vi "EyeSeeCam Plugin.vi"(10 "DC File":path, 11 "Data IN":T3={"Impulse Positions"=[{"Start"=395, "End"=549, "Impulse Plane"=enum."RALP", "Impulse Direction +ve?"=FALSE, "Time offset"=0, "Amplitude offset"=0.0}, {"Start"=603, "End"=760, "Impulse Plane"=enum."RALP", "Impulse Direction +ve?"=TRUE, "Time offset"=0, "Amplitude offset"=0.0}, {"Start"=785, "End"=938, "Impulse Plane"=enum."RALP", "Impulse Direction +ve?"=FALSE, "Time offset"=0, "Amplitude offset"=0.0}, {"Start"=980, "End"=1125, "Impulse Plane"=enum."LARP", "Impulse Direction +ve?"=FALSE, "Time offset"=0, "Amplitude offset"=0.0}, {"Start"=1179, "End"=1334, "Impulse Plane"=enum."LARP", "Impulse Direction +ve?"=TRUE, "Time offset"=0, "Amplitude offset"=0.0}, {"Start"=1723, "End"=1964, "Impulse Plane"=enum."Yaw", "Impulse Direction +ve?"=TRUE, "Time offset"=0, "Amplitude offset"=0.0}, {"Start"=1768, "End"=1968, "Impulse Plane"=enum."Yaw", "Impulse Direction +ve?"=TRUE, "Time offset"=0, "Amplitude offset"=0.0}, {"Start"=1812, "End"=1968, "Impulse Plane"=enum."Yaw", "Impulse Direction +ve?"=TRUE, "Time offset"=0, "Amplitude offset"=0.0}, {"Start"=4250, "End"=4393, "Impulse Plane"=enum."LARP", "Impulse Direction +ve?"=FALSE, "Time offset"=0, "Amplitude offset"=0.0}, {"Start"=4924, "End"=5072, "Impulse Plane"=enum."LARP", "Impulse Direction +ve?"=TRUE, "Time offset"=0, "Amplitude offset"=0.0}, {"Start"=5574, "End"=5721, "Impulse Plane"=enum."LARP", "Impulse Direction +ve?"=TRUE, "Time offset"=0, "Amplitude offset"=0.0}, {"Start"=6339, "End"=6491, "Impulse Plane"=enum."LARP", "Impulse Direction +ve?"=TRUE, "Time offset"=0, "Amplitude offset"=0.0}, {"Start"=6822, "End"=6967, "Impulse Plane"=enum."LARP", "Impulse Direction +ve?"=FALSE, "Time offset"=0, "Amplitude offset"=0.0}, {"Start"=7544, "End"=7701, "Impulse Plane"=enum."Pitch", "Impulse Direction +ve?"=TRUE, "Time offset"=0, "Amplitude offset"=0.0}, {"Start"=7928, "End"=8074, "Impulse Plane"=enum."LARP", "Impulse Direction +ve?"=TRUE, "Time offset"=0, "Amplitude offset"=0.0}, {"Start"=8313, "End"=8457, "Impulse Plane"=enum."LARP", "Impulse Direction +ve?"=FALSE, "Time offset"=0, "Amplitude offset"=0.0}, {"Start"=8807, "End"=8955, "Impulse Plane"=enum."LARP", "Impulse Direction +ve?"=FALSE, "Time offset"=0, "Amplitude offset"=0.0}, {"Start"=9308, "End"=9448, "Impulse Plane"=enum."LARP", "Impulse Direction +ve?"=FALSE, "Time offset"=0, "Amplitude offset"=0.0}, {"Start"=9758, "End"=9906, "Impulse Plane"=enum."LARP", "Impulse Direction +ve?"=TRUE, "Time offset"=0, "Amplitude offset"=0.0}, {"Start"=10165, "End"=10313, "Impulse Plane"=enum."LARP", "Impulse Direction +ve?"=TRUE, "Time offset"=0, "Amplitude offset"=0.0}, {"Start"=10605, "End"=10742, "Impulse Plane"=enum."LARP", "Impulse Direction +ve?"=FALSE, "Time offset"=0, "Amplitude offset"=0.0}, {"Start"=11345, "End"=11503, "Impulse Plane"=enum."Yaw", "Impulse Direction +ve?"=FALSE, "Time offset"=0, "Amplitude offset"=0.0}, {"Start"=12238, "End"=12394, "Impulse Plane"=enum."Yaw", "Impulse Direction +ve?"=FALSE, "Time offset"=0, "Amplitude offset"=0.0}, {"Start"=12374, "End"=12517, "Impulse Plane"=enum."LARP", "Impulse Direction +ve?"=FALSE, "Time offset"=0, "Amplitude offset"=0.0}, {"Start"=12860, "End"=13002, "Impulse Plane"=enum."LARP", "Impulse Direction +ve?"=TRUE, "Time offset"=0, "Amplitude offset"=0.0}, {"Start"=13499, "End"=13642, "Impulse Plane"=enum."LARP", "Impulse Direction +ve?"=FALSE, "Time offset"=0, "Amplitude offset"=0.0}, {"Start"=13998, "End"=14150, "Impulse Plane"=enum."LARP", "Impulse Direction +ve?"=TRUE, "Time offset"=0, "Amplitude offset"=0.0}, {"Start"=15617, "End"=15763, "Impulse Plane"=enum."LARP", "Impulse Direction +ve?"=FALSE, "Time offset"=0, "Amplitude offset"=0.0}], "No. Imp"=1, "Parameter Time Series"=[{"time offset"=0.0, "Offset"=0.0, "Gain"=1.0, "inverse"=FALSE, "filter data"=FALSE, "dots"=FALSE, "interpolate"=FALSE, "List 1"=1, "Color Box"=65295, "Boolean"=TRUE}, {"time offset"=0.0, "Offset"=0.0, "Gain"=1.0, "inverse"=FALSE, "filter data"=FALSE, "dots"=FALSE, "interpolate"=FALSE, "List 1"=13, "Color Box"=29695, "Boolean"=TRUE}], "Parameter Impuls Series"=[{"Color"=4652800, "Visible"=TRUE, "Channel"=7, "Invert"=FALSE, "Desaccade"=FALSE, "Offset"=0.0, "Gain"=1.0}, {"Color"=16860, "Visible"=TRUE, "Channel"=15, "Invert"=FALSE, "Desaccade"=FALSE, "Offset"=0.0, "Gain"=1.0}], "Experiment Parameters"={"Freq"=0.1, "Vel"=30, "Acc"=6000, "Stimulus"="HIT-RALP"}, "Autosort File"=refnum, "Data File"={"Data Channels"=array24x17202[412848 elements], "Sample Rate"=221, "Channel List"=["-", "Hz Velocity-in-Head", "-", "Hy Velocity-in-Head", "-", "Hx Velocity-in-Head", "Hl Velocity-in-Head", "Hr Velocity-in-Head", "-", "-", "-", "Lx Velocity-in-Head", "Ly Velocity-in-Head", "Lz Velocity-in-Head", "Ll Velocity-in-Head", "Lr Velocity-in-Head", "-", "-", "-", "Rx Velocity-in-Head", "Ry Velocity-in-Head", "Rz Velocity-in-Head", "Rl Velocity-in-Head", "Rr Velocity-in-Head"]}, "Experiment data path"=path "T:/50 _ HRC_DATA/Test Data/Vertical Canal VOG test", "Image data path"=path "C:/Users/w.figtree/Desktop", "LVS data path"=path "/Macintosh HD/Users/patrick/Studium/Diploma Thesis/Data Analysis", "Raw copy path"=path "/Macintosh HD/Users/patrick/Studium/Diploma Thesis/Data Analysis", "filename"="p00251s001e016c004t001.mat", "desaccading parameters"={"Tolerance"=3, "Acc Range"=7000.0, "Sample Rate"=221, "Impulse Plane 2"=enum."RALP", "Impulse dir"=TRUE}, "Experiment Parameters 2"={"Subject"="V Canal Test ", "Strain"="(2) _ vVOR", "Rotation plane"="YAW", "Experimenter"="Musterdoc", "Trial"=1.0, "Time"=8.0}, "Excel"={"Excel._Application"=refnum, "Use Excel"=TRUE, "Worksheet SINE"=refnum, "Row SINE"=0, "Worksheet TRANS"=refnum, "Row TRANS"=0}, "Session Config File"=refnum, "Autosort Parameter Set"=10, "EMA Version"="EMA 2011b", "desacc "={"Threshold 1 [Acc]"=7000.0, "Threshold 2 [% of TH1]"=60, "tolerance"=3, "Search WD "=0.1, " always use TH2"=FALSE, "Range"=3.0, "Max time"=120.0, "Min time"=20.0, "Velocity Threshold"=150}, "Cycle Nr for Saccades"={"POS"=0, "NEG"=3}, "calibration name"="No file selected"} {"Parameter Time Series"."time offset" format="%.3f"; "Parameter Time Series"."Gain" format="%.1f"; "Parameter Time Series"."Offset" format="%.1f"; "Parameter Time Series"."List 1" items=["Motor-Pos", "Motor-Vel", "Lx Position-in-Head", "Ly Position-in-Head", "Lz Position-in-Head", "Lx Velocity-in-Head", "Ly Velocity-in-Head", "Lz Velocity-in-Head", "Ll Velocity-in-Head", "Lr Velocity-in-Head", "Lx Accel-in-Head", "Ly Accel-in-Head", "Lz Accel-in-Head", "Rx Position-in-Head", "Ry Position-in-Head", "Rz Position-in-Head", "Rx Velocity-in-Head", "Ry Velocity-in-Head", "Rz Velocity-in-Head", "Rl Velocity-in-Head", "Rr Velocity-in-Head", "Rx Accel-in-Head", "Ry Accel-in-Head", "Rz Accel-in-Head", "Global Trigger", "", "", ""]; "Parameter Impuls Series"."Gain" format="%.1f"; "Parameter Impuls Series"."Offset" format="%.1f"}) -> (2 "Cancelled":bool, 3 "Data OUT":T3={"Impulse Positions"=[{"Start"=395, "End"=549, "Impulse Plane"=enum."RALP", "Impulse Direction +ve?"=FALSE, "Time offset"=0, "Amplitude offset"=0.0}, {"Start"=603, "End"=760, "Impulse Plane"=enum."RALP", "Impulse Direction +ve?"=TRUE, "Time offset"=0, "Amplitude offset"=0.0}, {"Start"=785, "End"=938, "Impulse Plane"=enum."RALP", "Impulse Direction +ve?"=FALSE, "Time offset"=0, "Amplitude offset"=0.0}, {"Start"=980, "End"=1125, "Impulse Plane"=enum."LARP", "Impulse Direction +ve?"=FALSE, "Time offset"=0, "Amplitude offset"=0.0}, {"Start"=1179, "End"=1334, "Impulse Plane"=enum."LARP", "Impulse Direction +ve?"=TRUE, "Time offset"=0, "Amplitude offset"=0.0}, {"Start"=1723, "End"=1964, "Impulse Plane"=enum."Yaw", "Impulse Direction +ve?"=TRUE, "Time offset"=0, "Amplitude offset"=0.0}, {"Start"=1768, "End"=1968, "Impulse Plane"=enum."Yaw", "Impulse Direction +ve?"=TRUE, "Time offset"=0, "Amplitude offset"=0.0}, {"Start"=1812, "End"=1968, "Impulse Plane"=enum."Yaw", "Impulse Direction +ve?"=TRUE, "Time offset"=0, "Amplitude offset"=0.0}, {"Start"=4250, "End"=4393, "Impulse Plane"=enum."LARP", "Impulse Direction +ve?"=FALSE, "Time offset"=0, "Amplitude offset"=0.0}, {"Start"=4924, "End"=5072, "Impulse Plane"=enum."LARP", "Impulse Direction +ve?"=TRUE, "Time offset"=0, "Amplitude offset"=0.0}, {"Start"=5574, "End"=5721, "Impulse Plane"=enum."LARP", "Impulse Direction +ve?"=TRUE, "Time offset"=0, "Amplitude offset"=0.0}, {"Start"=6339, "End"=6491, "Impulse Plane"=enum."LARP", "Impulse Direction +ve?"=TRUE, "Time offset"=0, "Amplitude offset"=0.0}, {"Start"=6822, "End"=6967, "Impulse Plane"=enum."LARP", "Impulse Direction +ve?"=FALSE, "Time offset"=0, "Amplitude offset"=0.0}, {"Start"=7544, "End"=7701, "Impulse Plane"=enum."Pitch", "Impulse Direction +ve?"=TRUE, "Time offset"=0, "Amplitude offset"=0.0}, {"Start"=7928, "End"=8074, "Impulse Plane"=enum."LARP", "Impulse Direction +ve?"=TRUE, "Time offset"=0, "Amplitude offset"=0.0}, {"Start"=8313, "End"=8457, "Impulse Plane"=enum."LARP", "Impulse Direction +ve?"=FALSE, "Time offset"=0, "Amplitude offset"=0.0}, {"Start"=8807, "End"=8955, "Impulse Plane"=enum."LARP", "Impulse Direction +ve?"=FALSE, "Time offset"=0, "Amplitude offset"=0.0}, {"Start"=9308, "End"=9448, "Impulse Plane"=enum."LARP", "Impulse Direction +ve?"=FALSE, "Time offset"=0, "Amplitude offset"=0.0}, {"Start"=9758, "End"=9906, "Impulse Plane"=enum."LARP", "Impulse Direction +ve?"=TRUE, "Time offset"=0, "Amplitude offset"=0.0}, {"Start"=10165, "End"=10313, "Impulse Plane"=enum."LARP", "Impulse Direction +ve?"=TRUE, "Time offset"=0, "Amplitude offset"=0.0}, {"Start"=10605, "End"=10742, "Impulse Plane"=enum."LARP", "Impulse Direction +ve?"=FALSE, "Time offset"=0, "Amplitude offset"=0.0}, {"Start"=11345, "End"=11503, "Impulse Plane"=enum."Yaw", "Impulse Direction +ve?"=FALSE, "Time offset"=0, "Amplitude offset"=0.0}, {"Start"=12238, "End"=12394, "Impulse Plane"=enum."Yaw", "Impulse Direction +ve?"=FALSE, "Time offset"=0, "Amplitude offset"=0.0}, {"Start"=12374, "End"=12517, "Impulse Plane"=enum."LARP", "Impulse Direction +ve?"=FALSE, "Time offset"=0, "Amplitude offset"=0.0}, {"Start"=12860, "End"=13002, "Impulse Plane"=enum."LARP", "Impulse Direction +ve?"=TRUE, "Time offset"=0, "Amplitude offset"=0.0}, {"Start"=13499, "End"=13642, "Impulse Plane"=enum."LARP", "Impulse Direction +ve?"=FALSE, "Time offset"=0, "Amplitude offset"=0.0}, {"Start"=13998, "End"=14150, "Impulse Plane"=enum."LARP", "Impulse Direction +ve?"=TRUE, "Time offset"=0, "Amplitude offset"=0.0}, {"Start"=15617, "End"=15763, "Impulse Plane"=enum."LARP", "Impulse Direction +ve?"=FALSE, "Time offset"=0, "Amplitude offset"=0.0}], "No. Imp"=1, "Parameter Time Series"=[{"time offset"=0.0, "Offset"=0.0, "Gain"=1.0, "inverse"=FALSE, "filter data"=FALSE, "dots"=FALSE, "interpolate"=FALSE, "List 1"=1, "Color Box"=65295, "Boolean"=TRUE}, {"time offset"=0.0, "Offset"=0.0, "Gain"=1.0, "inverse"=FALSE, "filter data"=FALSE, "dots"=FALSE, "interpolate"=FALSE, "List 1"=13, "Color Box"=29695, "Boolean"=TRUE}], "Parameter Impuls Series"=[{"Color"=4652800, "Visible"=TRUE, "Channel"=1, "Invert"=FALSE, "Desaccade"=FALSE, "Offset"=0.0, "Gain"=1.0}, {"Color"=16860, "Visible"=TRUE, "Channel"=13, "Invert"=FALSE, "Desaccade"=FALSE, "Offset"=0.0, "Gain"=1.0}], "Experiment Parameters"={"Freq"=0.1, "Vel"=30, "Acc"=6000, "Stimulus"="HIT-LARP"}, "Autosort File"=refnum, "Data File"={"Data Channels"=array24x20058[481392 elements], "Sample Rate"=221, "Channel List"=["-", "Hz Velocity-in-Head", "-", "Hy Velocity-in-Head", "-", "Hx Velocity-in-Head", "Hl Velocity-in-Head", "Hr Velocity-in-Head", "-", "-", "-", "Lx Velocity-in-Head", "Ly Velocity-in-Head", "Lz Velocity-in-Head", "Ll Velocity-in-Head", "Lr Velocity-in-Head", "-", "-", "-", "Rx Velocity-in-Head", "Ry Velocity-in-Head", "Rz Velocity-in-Head", "Rl Velocity-in-Head", "Rr Velocity-in-Head"]}, "Experiment data path"=path "T:/50 _ HRC_DATA/Test Data/Vertical Canal VOG test", "Image data path"=path "C:/Users/w.figtree/Desktop", "LVS data path"=path "/Macintosh HD/Users/patrick/Studium/Diploma Thesis/Data Analysis", "Raw copy path"=path "/Macintosh HD/Users/patrick/Studium/Diploma Thesis/Data Analysis", "filename"="p00251s001e016c005t001.mat", "desaccading parameters"={"Tolerance"=3, "Acc Range"=7000.0, "Sample Rate"=221, "Impulse Plane 2"=enum."RALP", "Impulse dir"=TRUE}, "Experiment Parameters 2"={"Subject"="V Canal Test ", "Strain"="(2) _ vVOR", "Rotation plane"="YAW", "Experimenter"="Musterdoc", "Trial"=1.0, "Time"=8.0}, "Excel"={"Excel._Application"=refnum, "Use Excel"=TRUE, "Worksheet SINE"=refnum, "Row SINE"=0, "Worksheet TRANS"=refnum, "Row TRANS"=0}, "Session Config File"=refnum, "Autosort Parameter Set"=10, "EMA Version"="EMA 2011b", "desacc "={"Threshold 1 [Acc]"=7000.0, "Threshold 2 [% of TH1]"=60, "tolerance"=3, "Search WD "=0.1, " always use TH2"=FALSE, "Range"=3.0, "Max time"=120.0, "Min time"=20.0, "Velocity Threshold"=150}, "Cycle Nr for Saccades"={"POS"=0, "NEG"=3}, "calibration name"="No file selected"} {"Parameter Time Series"."time offset" format="%.3f"; "Parameter Time Series"."Gain" format="%.1f"; "Parameter Time Series"."Offset" format="%.1f"; "Parameter Time Series"."List 1" items=["Motor-Pos", "Motor-Vel", "Lx Position-in-Head", "Ly Position-in-Head", "Lz Position-in-Head", "Lx Velocity-in-Head", "Ly Velocity-in-Head", "Lz Velocity-in-Head", "Ll Velocity-in-Head", "Lr Velocity-in-Head", "Lx Accel-in-Head", "Ly Accel-in-Head", "Lz Accel-in-Head", "Rx Position-in-Head", "Ry Position-in-Head", "Rz Position-in-Head", "Rx Velocity-in-Head", "Ry Velocity-in-Head", "Rz Velocity-in-Head", "Rl Velocity-in-Head", "Rr Velocity-in-Head", "Rx Accel-in-Head", "Ry Accel-in-Head", "Rz Accel-in-Head", "Global Trigger", "", "", ""]; "Parameter Impuls Series"."Gain" format="%.1f"; "Parameter Impuls Series"."Offset" format="%.1f"})   [LabVIEW 2016]
uses:
  core/type-defs/TD_Statemachine-Data.ctl
  core/type-defs/TD_Time Series.ctl
  core/type-defs/TD_Impulse Parameter.ctl
  core/core.lvlib
panel:
  out "Process Error":errorcluster
  in  "BTN_Process":bool
  in  "Tab Control":enum32{"Settings", "Time Plot", "Impulse Plot"}(tab)
  in  "Btn_ZeroGyro":bool
  in  "alignPR?":bool caption="Align Head pitch/roll axes?"
  in  "manualGOff?":bool caption="Use manual gyro offset?"
  in  "Yaw":dbl caption="Yaw (dps)"
  in  "Pitch":dbl caption="Pitch (dps)"
  in  "Roll":dbl caption="Roll (dps)"
  in  "Head Calibration File":path
  in  "Data File":path
  in  "Eye Calibration File":path
  in  "eyeFromPx?":bool=TRUE caption="Calculate eye data from pupil centroid?"
  in  "Time Plot Selection":T1=[{"time offset"=0.0, "Offset"=0.0, "Gain"=1.0, "inverse"=FALSE, "filter data"=FALSE, "dots"=FALSE, "interpolate"=FALSE, "List 1"=1, "Color Box"=65295, "Boolean"=TRUE}, {"time offset"=0.0, "Offset"=0.0, "Gain"=1.0, "inverse"=FALSE, "filter data"=FALSE, "dots"=FALSE, "interpolate"=FALSE, "List 1"=3, "Color Box"=16717731, "Boolean"=FALSE}, {"time offset"=0.0, "Offset"=0.0, "Gain"=1.0, "inverse"=FALSE, "filter data"=FALSE, "dots"=FALSE, "interpolate"=FALSE, "List 1"=6, "Color Box"=16742144, "Boolean"=FALSE}, {"time offset"=0.0, "Offset"=0.0, "Gain"=1.0, "inverse"=FALSE, "filter data"=FALSE, "dots"=FALSE, "interpolate"=FALSE, "List 1"=7, "Color Box"=14419712, "Boolean"=FALSE}, {"time offset"=0.0, "Offset"=0.0, "Gain"=1.0, "inverse"=FALSE, "filter data"=FALSE, "dots"=FALSE, "interpolate"=FALSE, "List 1"=13, "Color Box"=16777224, "Boolean"=TRUE}, {"time offset"=0.0, "Offset"=0.0, "Gain"=1.0, "inverse"=FALSE, "filter data"=FALSE, "dots"=FALSE, "interpolate"=FALSE, "List 1"=12, "Color Box"=2298623, "Boolean"=FALSE}] {"time offset" format="%.3f"; "Gain" format="%.1f"; "Offset" format="%.1f"; "List 1" items=["-", "Hz Velocity-in-Head", "-", "Hy Velocity-in-Head", "-", "Hx Velocity-in-Head", "Hl Velocity-in-Head", "Hr Velocity-in-Head", "-", "Ly Position-in-Head", "Lz Position-in-Head", "-", "Ly Velocity-in-Head", "Lz Velocity-in-Head", "-", "-", "-", "-", "-", "-", "-", "-", "-", "-"]}
  in  "Impulse Plot Selection":T2=[{"Color"=4652800, "Visible"=TRUE, "Channel"=1, "Invert"=FALSE, "Desaccade"=FALSE, "Offset"=0.0, "Gain"=1.0}, {"Color"=16717731, "Visible"=FALSE, "Channel"=3, "Invert"=FALSE, "Desaccade"=FALSE, "Offset"=0.0, "Gain"=1.0}, {"Color"=16742144, "Visible"=FALSE, "Channel"=6, "Invert"=FALSE, "Desaccade"=FALSE, "Offset"=0.0, "Gain"=1.0}, {"Color"=14419712, "Visible"=FALSE, "Channel"=7, "Invert"=FALSE, "Desaccade"=FALSE, "Offset"=0.0, "Gain"=1.0}, {"Color"=16777224, "Visible"=TRUE, "Channel"=13, "Invert"=FALSE, "Desaccade"=FALSE, "Offset"=0.0, "Gain"=1.0}, {"Color"=2298623, "Visible"=FALSE, "Channel"=12, "Invert"=FALSE, "Desaccade"=FALSE, "Offset"=0.0, "Gain"=1.0}] {"Gain" format="%.1f"; "Offset" format="%.1f"; "Channel" items=["-", "Hz Velocity-in-Head", "-", "Hy Velocity-in-Head", "-", "Hx Velocity-in-Head", "Hl Velocity-in-Head", "Hr Velocity-in-Head", "-", "Ly Position-in-Head", "Lz Position-in-Head", "-", "Ly Velocity-in-Head", "Lz Velocity-in-Head", "-", "-", "-", "-", "-", "-", "-", "-", "-", "-"]}
  # "Specify a file for analysis..."
  # "Offset    Gain       Inv                     Channel                       Col   Vis  Sac"
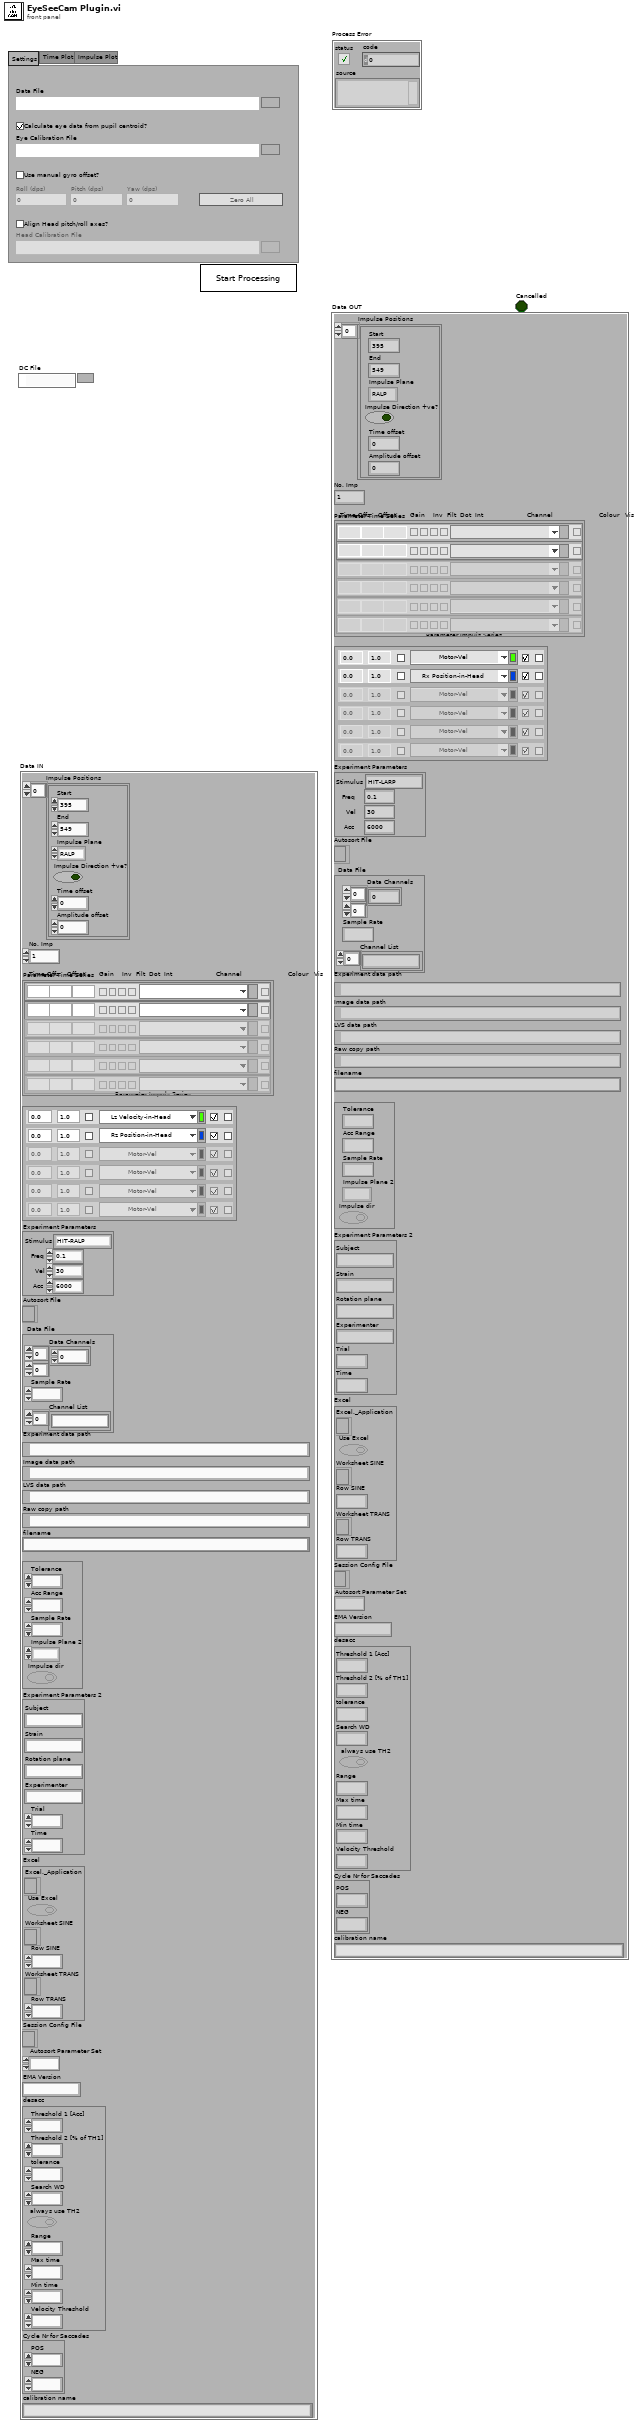
[diagram p1: front panel]
types:
  T1 = typedef "core.lvlib/TD_Time Series.ctl" = cluster{"time offset":dbl, "Offset":dbl, "Gain":dbl, "inverse":bool, "filter data":bool, "dots":bool, "interpolate":bool, "List 1":u16, "Color Box":u32, "Boolean":bool}[]
  T2 = typedef "core.lvlib/TD_Impulse Parameter.ctl" = cluster{"Color":u32, "Visible":bool, "Channel":u16, "Invert":bool, "Desaccade":bool, "Offset":dbl, "Gain":dbl}[]
  T3 = typedef "core.lvlib/TD_Statemachine-Data.ctl" = cluster{"Impulse Positions":cluster{"Start":i32, "End":i32, "Impulse Plane":enum16{"Other", "Yaw", "Pitch", "Roll", "LARP", "RALP"}, "Impulse Direction +ve?":bool, "Time offset":i32, "Amplitude offset":dbl}[], "No. Imp":i32, "Parameter Time Series":T1, "Parameter Impuls Series":T2, "Experiment Parameters":cluster{"Freq":dbl, "Vel":i32, "Acc":i32, "Stimulus":string}, "Autosort File":refnum<file>, "Data File":cluster{"Data Channels":dbl[][], "Sample Rate":i32, "Channel List":string[]}, "Experiment data path":path, "Image data path":path, "LVS data path":path, "Raw copy path":path, "filename":string, "desaccading parameters":cluster{"Tolerance":i32, "Acc Range":dbl, "Sample Rate":i32, "Impulse Plane 2":enum16{"Other", "Yaw", "Pitch", "Roll", "LARP", "RALP"}, "Impulse dir":bool}, "Experiment Parameters 2":cluster{"Subject":string, "Strain":string, "Rotation plane":string, "Experimenter":string, "Trial":dbl, "Time":dbl}, "Excel":cluster{"Excel._Application":refnum<k7>, "Use Excel":bool, "Worksheet SINE":refnum<k7>, "Row SINE":i32, "Worksheet TRANS":refnum<k7>, "Row TRANS":i32}, "Session Config File":refnum<file>, "Autosort Parameter Set":i32, "EMA Version":string, "desacc ":cluster{"Threshold 1 [Acc]":dbl, "Threshold 2 [% of TH1]":i32, "tolerance":i32, "Search WD ":dbl, " always use TH2":bool, "Range":dbl, "Max time":dbl, "Min time":dbl, "Velocity Threshold":i32}, "Cycle Nr for Saccades":cluster{"POS":i32, "NEG":i32}, "calibration name":string}
  T4 = enum8{"Enabled", "Disabled", "Disabled and Grayed Out"}
  T5 = cluster{"time offset":dbl, "Offset":dbl, "Gain":dbl, "inverse":bool, "filter data":bool, "dots":bool, "interpolate":bool, "List 1":u16, "Color Box":u32, "Boolean":bool}
  T6 = cluster{"Color":u32, "Visible":bool, "Channel":u16, "Invert":bool, "Desaccade":bool, "Offset":dbl, "Gain":dbl}
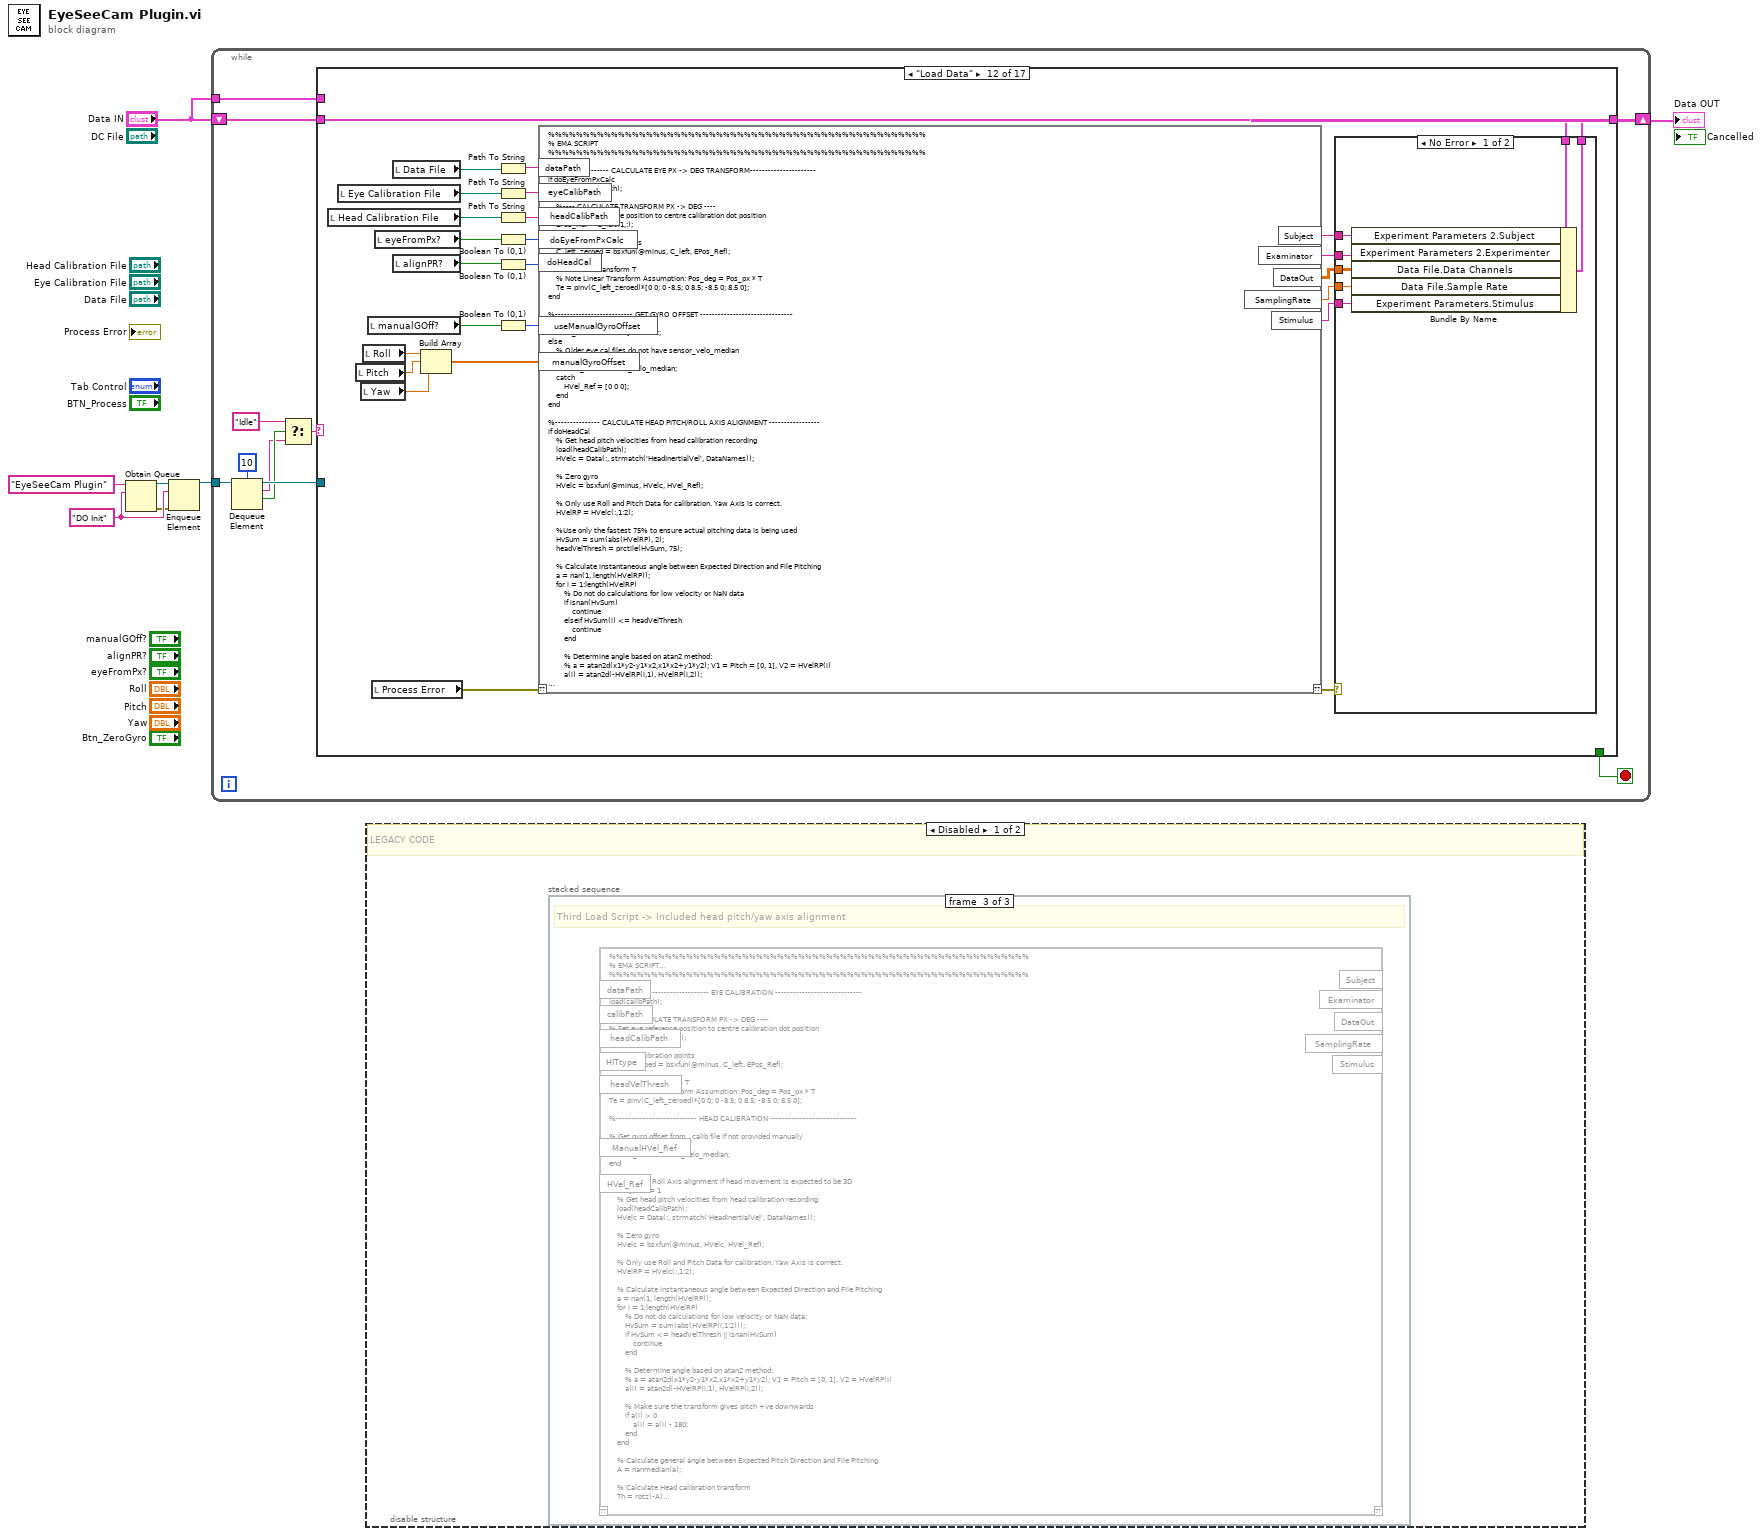
[diagram p0: block diagram]
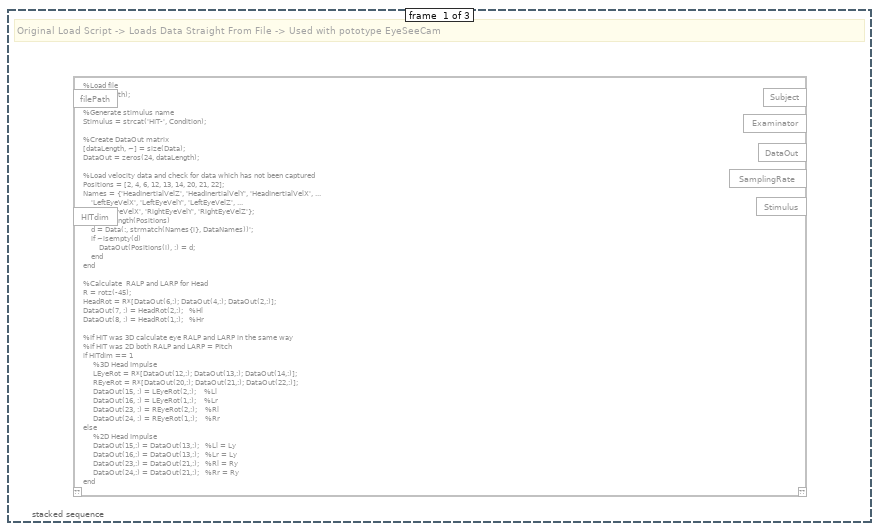
[diagram p2: hidden frame]
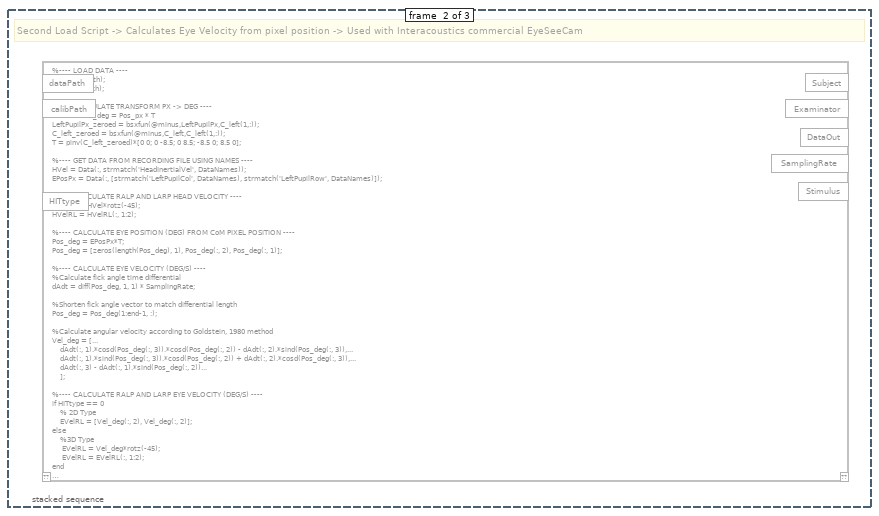
[diagram p3: hidden frame]
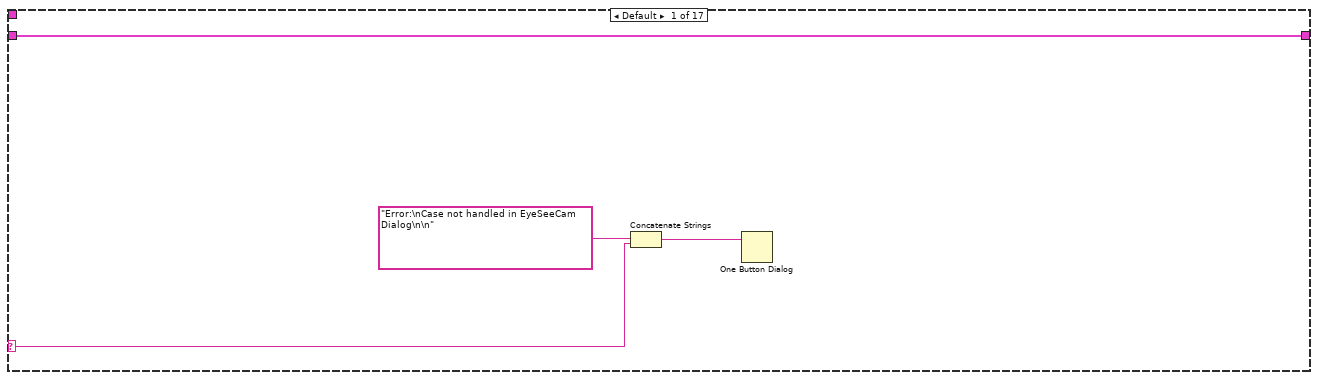
[diagram p5: hidden frame]
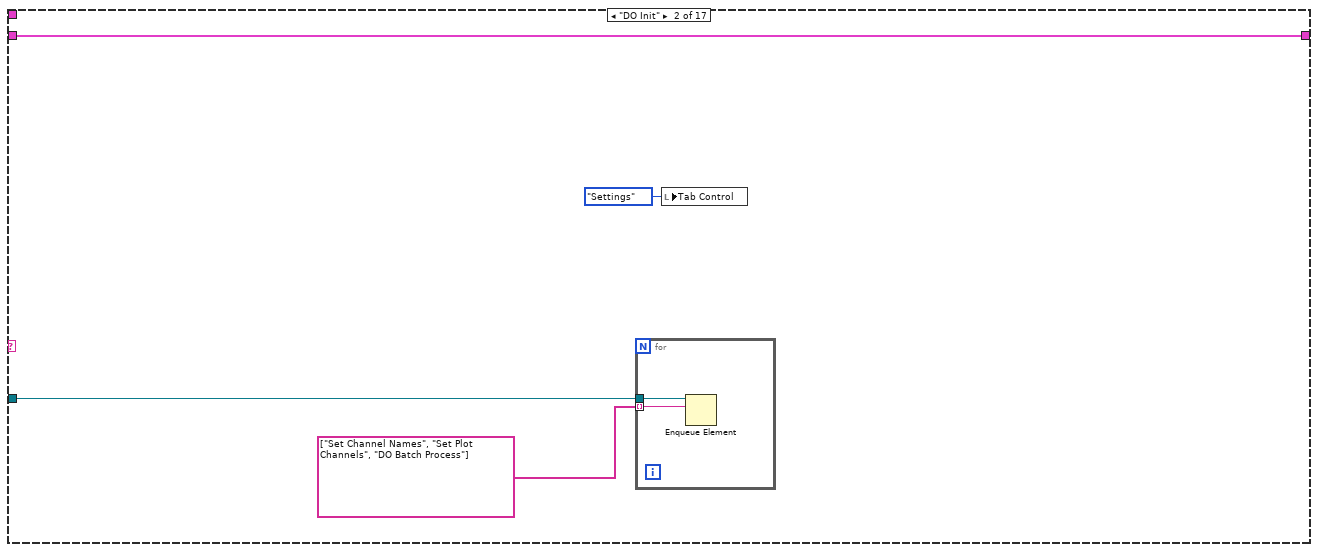
[diagram p6: hidden frame]
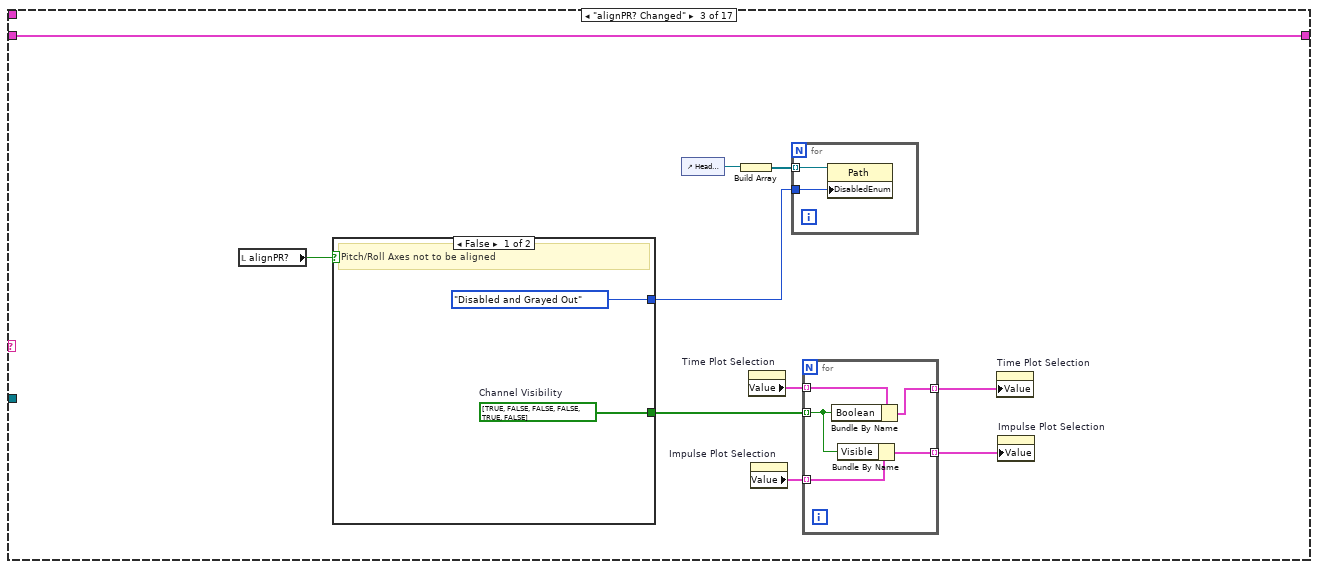
[diagram p7: hidden frame]
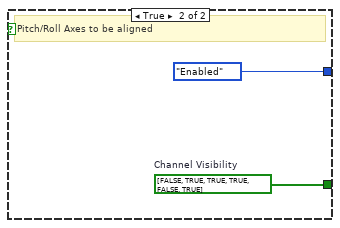
[diagram p8: hidden frame]
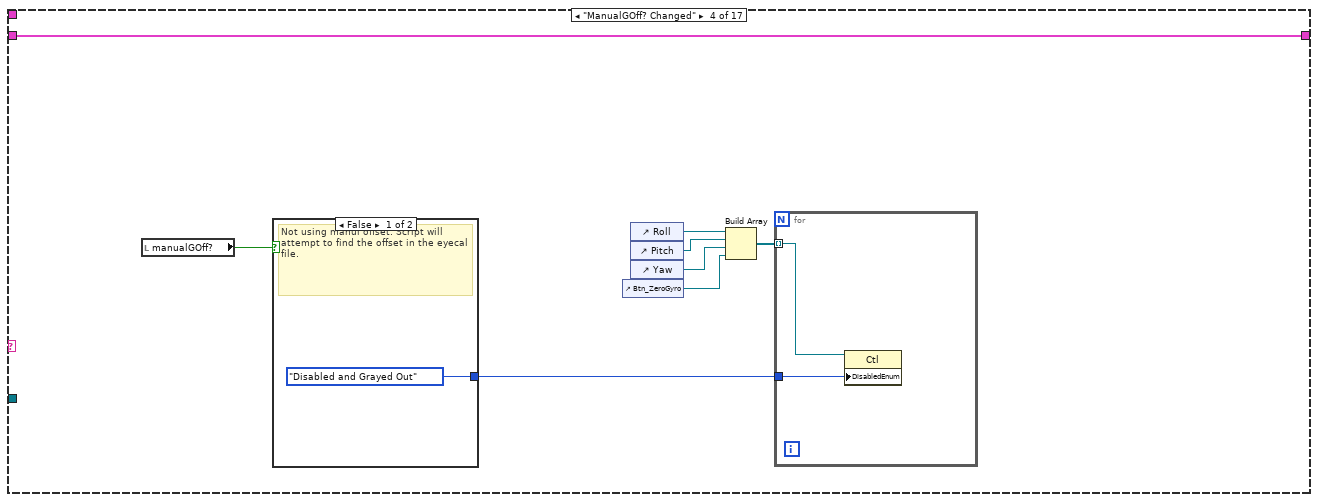
[diagram p9: hidden frame]
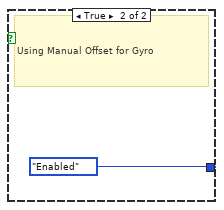
[diagram p10: hidden frame]
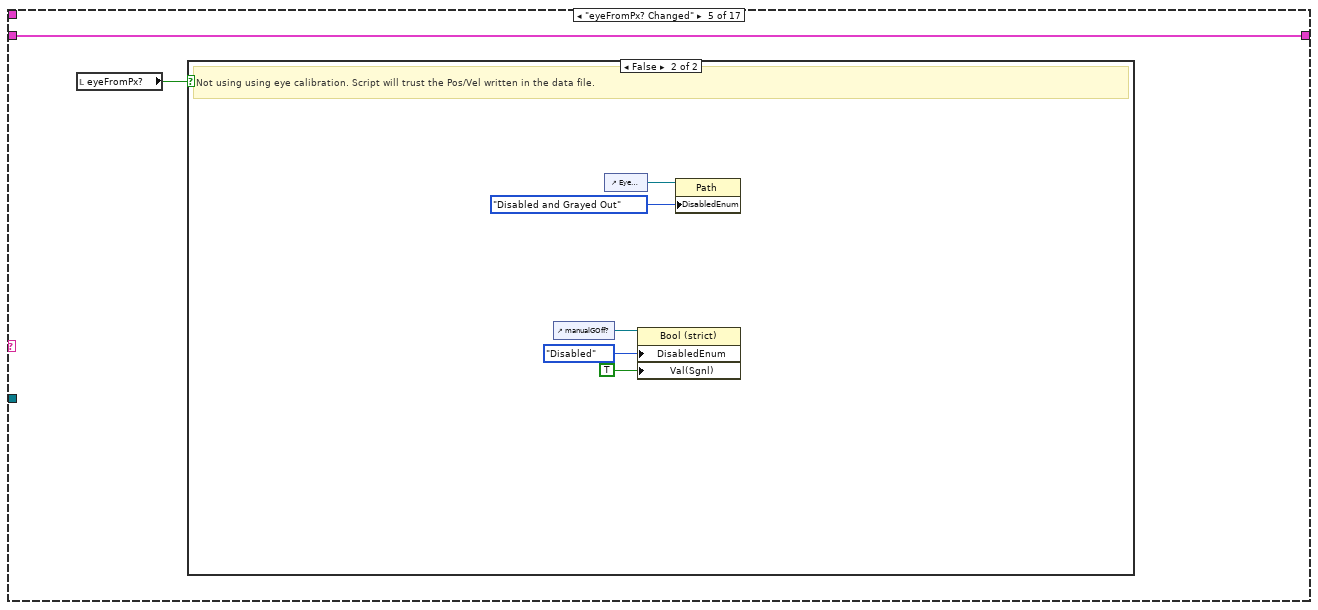
[diagram p11: hidden frame]
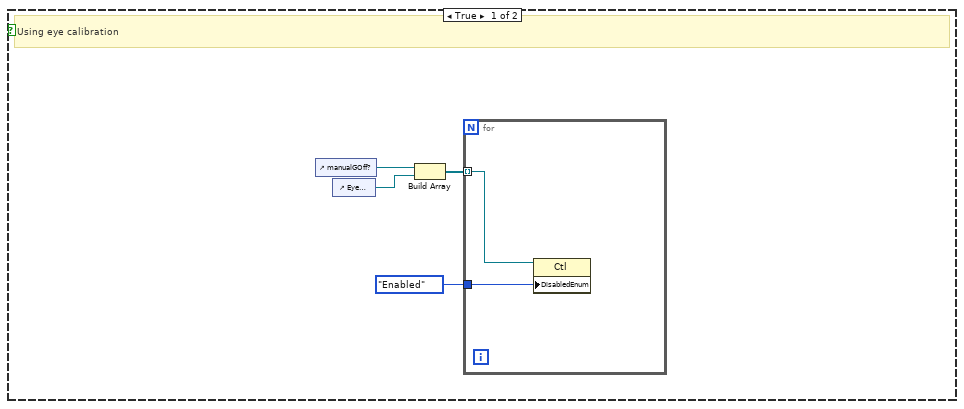
[diagram p12: hidden frame]
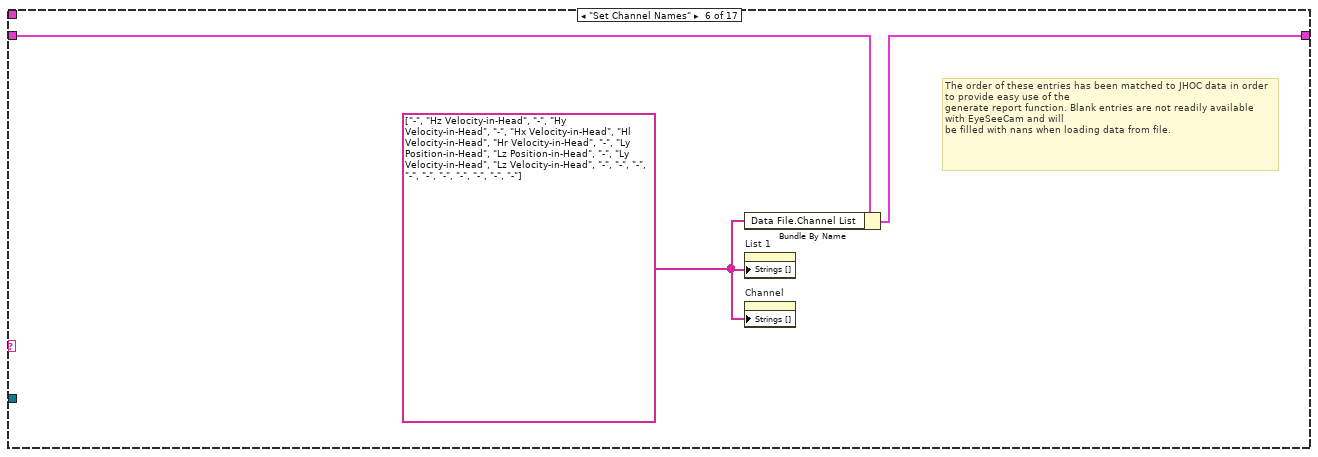
[diagram p13: hidden frame]
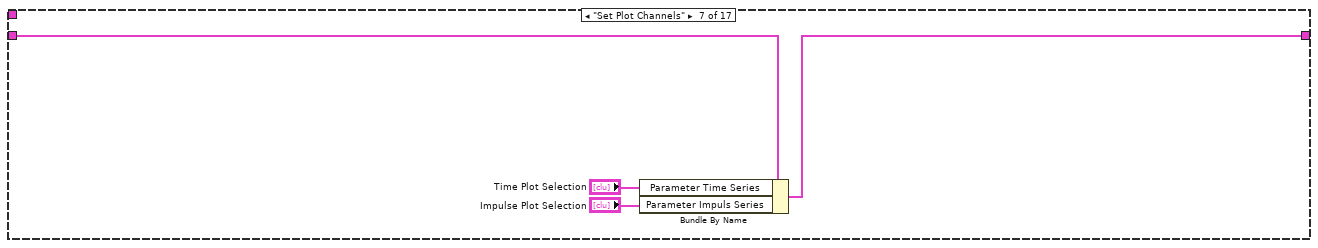
[diagram p14: hidden frame]
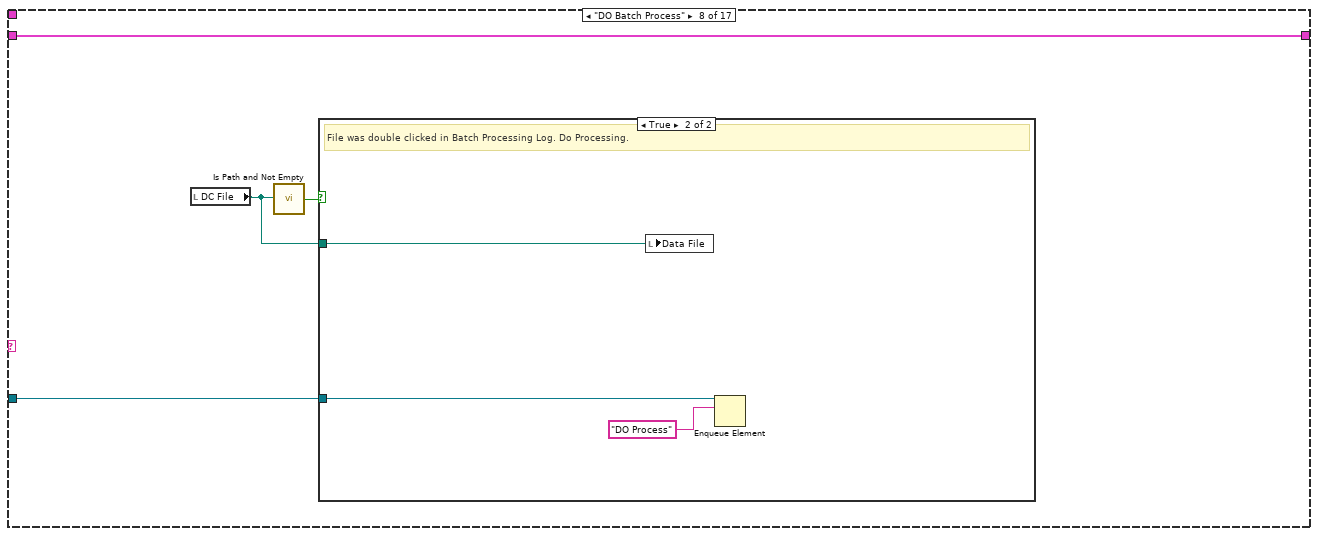
[diagram p15: hidden frame]
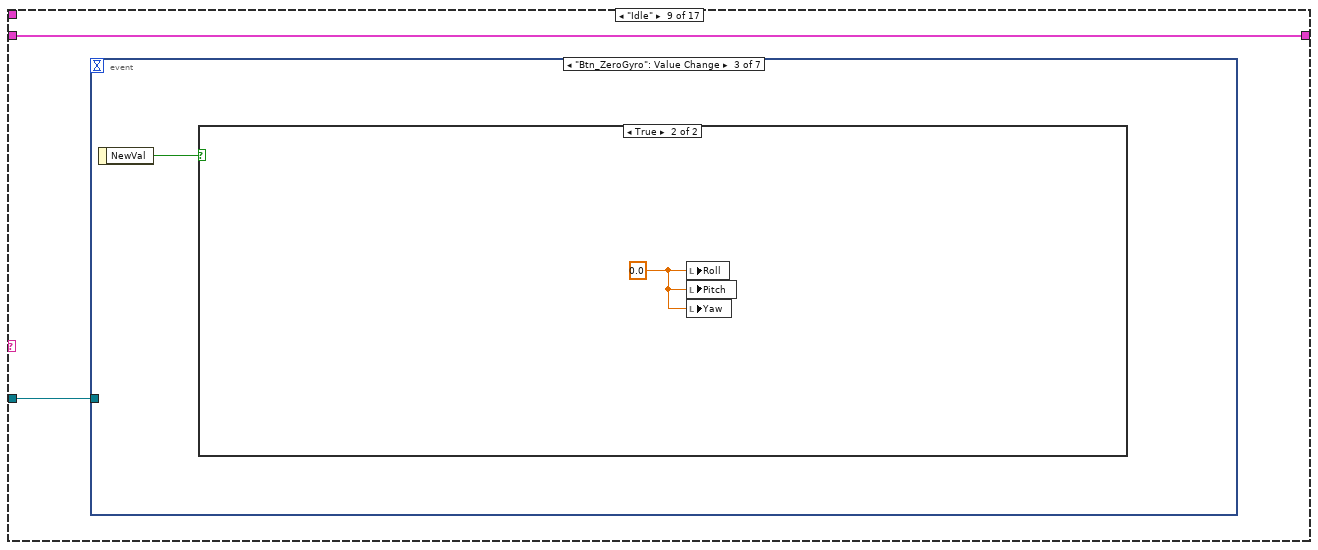
[diagram p17: hidden frame]
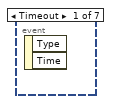
[diagram p18: hidden frame]
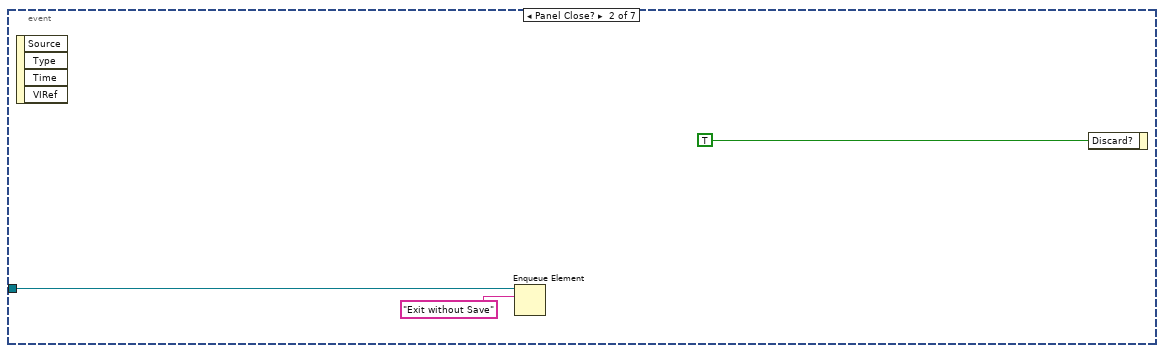
[diagram p19: hidden frame]
diagram:
  w5 = "DO Init" ("name (unnamed)")
  n1 = Obtain Queue(name (unnamed)="EyeSeeCam Plugin", element data type=w5) -> (queue out=w6:refnum<queue>, error out=w4:errorcluster)  [unwired: 3 in, 1 out]
  n2 = Enqueue Element(queue=w6, element=w5, error in (no error)=w4) -> (queue out=w3:refnum<queue>)  [unwired: 1 in, 2 out]
  n3 = while {
    tunnel: w3 -> [w18]
    shift-right: [w16] -> w2
    shift-left: "Data IN" -> [w17]
    tunnel: "Data IN" -> [w13]
    stop <- w14 stop-if-true
    n4 = Dequeue Element(queue=w18, timeout in ms (-1)=10) -> (queue out=w15:refnum<queue>, element=w11:string, timed out?=w12:bool)  [unwired: 1 in, 1 out]
    n5 = Select(t="Idle", s=w12, f=w11) -> (s? t:f=w9:string)
    n6 = case shown="\"Load Data\"" w9 {
      selector: w9 -> [w20 _ _ _ _ _ _ _ _ _ _ _ _ _ _ _ _]
      tunnel: w17 -> [w22 w26 w38 w57 w63 w77 w81 w84 w90 w109 w113 w137 w164 w178 w181 w197 _]
      tunnel: [w22 w26 w38 w57 w63 w76 w80 w84 w90 w109 w113 w136 w163 w178 w181 w197 w201] -> w16
      tunnel: w15 -> [_ w25 _ _ _ _ _ w85 w89 w108 _ _ _ w174 _ _ _]
      tunnel: [_ _ _ _ _ _ _ _ _ _ _ _ _ _ _ TRUE TRUE] -> w14
      tunnel: w13 -> [_ _ _ _ _ _ _ _ _ _ _ _ _ _ _ _ w201]
      frame Default {
        n7 = Concatenate Strings("Error:\nCase not handled in EyeSeeCam Dialog\n\n" ("message"), w20) -> (w19:string)
        n8 = One Button Dialog(message=w19) -> ()  [unwired: 1 in, 1 out]
      }
      frame "DO Init" {
        n9 = for {
          tunnel: w25 -> [w28]
          tunnel: string[] ["Set Channel Names", "Set Plot Channels", "DO Batch Process"] -> [w27] mode=indexing
          n10 = Enqueue Element(queue=w28, element=w27) -> ()  [unwired: 2 in, 3 out]
        }
        n11 = local write "Tab Control"(enum32{"Settings", "Time Plot", "Impulse Plot"}."Settings" ("Tab Control")) -> ()
      }
      frame "alignPR? Changed" {
        n12 = local read "alignPR?"() -> (w37:bool)
        n13 = case shown="False" w37 {
          tunnel: [T4."Disabled and Grayed Out" ("Disabled") T4."Enabled" ("Disabled")] -> w29
          tunnel: [w46 w48] -> w35
          frame False {
            w46 = bool[] [TRUE, FALSE, FALSE, FALSE, TRUE, FALSE]  # Channel Visibility
            # "Pitch/Roll Axes not to be aligned"
          }
          frame True {
            w48 = bool[] [FALSE, TRUE, TRUE, TRUE, FALSE, TRUE]  # Channel Visibility
            # "Pitch/Roll Axes to be aligned"
          }
        }
        n14 = control-ref of="Head Calibration File"() -> (w31:refnum<vi>)
        n15 = Build Array(w31) -> (w30:refnum<vi>[])
        n16 = property on="Time Plot Selection" class="Arr (strict)"() -> ("Value"=w36:T1)  [unwired: 2 in, 2 out]
        n17 = property on="Impulse Plot Selection" class="Arr (strict)"() -> ("Value"=w33:T2)  [unwired: 2 in, 2 out]
        n18 = for {
          tunnel: w30 -> [w40] mode=indexing
          tunnel: w29 -> [w39]
          n19 = property class="Path"(reference=w40, "DisabledEnum"=w39) -> ()  [unwired: 1 in, 2 out]
        }
        n20 = for {
          tunnel: w36 -> [w45] mode=indexing
          tunnel: [w44] -> w34 mode=indexing
          tunnel: w35 -> [w41] mode=indexing
          tunnel: w33 -> [w43] mode=indexing
          tunnel: [w42] -> w32 mode=indexing
          n21 = Bundle By Name(cluster=w45, "Boolean"=w41) -> (w44:T5)
          n22 = Bundle By Name(cluster=w43, "Visible"=w41) -> (w42:T6)
        }
        n23 = property on="Time Plot Selection" class="Arr (strict)"("Value"=w34) -> ()  [unwired: 2 in, 2 out]
        n24 = property on="Impulse Plot Selection" class="Arr (strict)"("Value"=w32) -> ()  [unwired: 2 in, 2 out]
      }
      frame "ManualGOff? Changed" {
        n25 = local read "manualGOff?"() -> (w56:bool)
        n26 = case shown="False" w56 {
          tunnel: [T4."Disabled and Grayed Out" ("Disabled") T4."Enabled" ("Disabled")] -> w51
          frame False {
            # "Not using manul offset. Script will attempt to find the offset in the eyecal file."
          }
          frame True {
            # "Using Manual Offset for Gyro"
          }
        }
        n27 = control-ref of="Btn_ZeroGyro"() -> (w50:refnum<vi>)
        n28 = control-ref of="Roll"() -> (w55:refnum<vi>)
        n29 = control-ref of="Pitch"() -> (w54:refnum<vi>)
        n30 = control-ref of="Yaw"() -> (w53:refnum<vi>)
        n31 = Build Array(w55, w54, w53, w50) -> (w52:refnum<vi>[])
        n32 = for {
          tunnel: w52 -> [w59] mode=indexing
          tunnel: w51 -> [w58]
          n33 = property class="Ctl"(reference=w59, "DisabledEnum"=w58) -> ()  [unwired: 1 in, 2 out]
        }
      }
      frame "eyeFromPx? Changed" {
        n34 = local read "eyeFromPx?"() -> (w62:bool)
        n35 = case shown="False" w62 {
          frame True {
            # "Using eye calibration"
            n36 = control-ref of="manualGOff?"() -> (w66:refnum<vi>)
            n37 = control-ref of="Eye Calibration File"() -> (w65:refnum<vi>)
            n38 = Build Array(w66, w65) -> (w67:refnum<vi>[])
            n39 = for {
              tunnel: w67 -> [w69] mode=indexing
              tunnel: T4."Enabled" ("Disabled") -> [w68]
              n40 = property class="Ctl"(reference=w69, "DisabledEnum"=w68) -> ()  [unwired: 1 in, 2 out]
            }
          }
          frame False {
            # "Not using using eye calibration. Script will trust the Pos/Vel written in the data file."
            n41 = control-ref of="manualGOff?"() -> (w72:refnum<vi>)
            n42 = control-ref of="Eye Calibration File"() -> (w73:refnum<vi>)
            n43 = property class="Bool (strict)"(reference=w72, "DisabledEnum"=T4."Disabled" ("Disabled"), "Val(Sgnl)"=TRUE ("Value")) -> ()  [unwired: 1 in, 2 out]
            n44 = property class="Path"(reference=w73, "DisabledEnum"=T4."Disabled and Grayed Out" ("Disabled")) -> ()  [unwired: 1 in, 2 out]
          }
        }
      }
      frame "Set Channel Names" {
        w75 = string[] ["-", "Hz Velocity-in-Head", "-", "Hy Velocity-in-Head", "-", "Hx Velocity-in-Head", "Hl Velocity-in-Head", "Hr Velocity-in-Head", "-", "Ly Position-in-Head", "Lz Position-in-Head", "-", "Ly Velocity-in-Head", "Lz Velocity-in-Head", "-", "-", "-", "-", "-", "-", "-", "-", "-", "-"]
        # "The order of these entries has been matched to JHOC data in order to provide easy use of the\ngenerate report function. Blank entries are not readily available with EyeSeeCam and will\nbe filled with nans when loading data from file."
        n45 = Bundle By Name(cluster=w77, "Data File.Channel List"=w75) -> (w76:T3)
        n46 = property on="List 1" class="Ring (strict)"("Strings []"=w75) -> ()  [unwired: 2 in, 2 out]
        n47 = property on="Channel" class="Ring (strict)"("Strings []"=w75) -> ()  [unwired: 2 in, 2 out]
      }
      frame "Set Plot Channels" {
        n48 = Bundle By Name(cluster=w81, "Parameter Time Series"="Time Plot Selection", "Parameter Impuls Series"="Impulse Plot Selection") -> (w80:T3)
      }
      frame "DO Batch Process" {
        n49 = local read "DC File"() -> (w83:path)
        n50 = call <vilib>:"Is Path and Not Empty.vi"("path"=w83) -> ("Is Path and Not Empty?"=w82:bool)  [unwired: 4 in]
        n51 = case shown="True" w82 {
          tunnel: w83 -> [_ w88]
          tunnel: w85 -> [_ w87]
          frame False {
            # "This dialog was not open by batch processing. Do nothing."
          }
          frame True {
            # "File was double clicked in Batch Processing Log. Do Processing."
            n52 = local write "Data File"(w88) -> ()
            n53 = Enqueue Element(queue=w87, element="DO Process") -> ()  [unwired: 2 in, 3 out]
          }
        }
      }
      frame "Idle" {
        n54 = event shown="[2] \"Btn_ZeroGyro\": Value Change" {
          selector: _ -> [_ _ _ _ _ _ _]
          dyn-events: _ -> [_ _ _ _ _ _ _]
          timeout: _ -> [_ _ _ _ _ _ _]
          tunnel: w89 -> [_ w91 _ w97 w98 w103 w105]
          event Timeout {
            n55 = event-data() -> ()  [unwired: 1 in, 2 out]
          }
          event Panel Close? {
            n56 = event-data() -> ()  [unwired: 1 in, 4 out]
            n57 = Enqueue Element(queue=w91, element="Exit without Save") -> ()  [unwired: 2 in, 3 out]
            n58 = event-data("Discard?"=TRUE) -> ()  [unwired: 1 in, 1 out]
          }
          event "Btn_ZeroGyro": Value Change {
            n59 = event-data() -> ("NewVal"=w94:bool)  [unwired: 1 in]
            n60 = case shown="True" w94 {
              frame False {
              }
              frame True {
                w95 = 0.0 ("Roll")
                n61 = local write "Roll"(w95) -> ()
                n62 = local write "Pitch"(w95) -> ()
                n63 = local write "Yaw"(w95) -> ()
              }
            }
          }
          event "BTN_Process": Mouse Down {
            n64 = event-data() -> ()  [unwired: 1 in, 7 out]
            n65 = Enqueue Element(queue=w97, element="DO Process") -> ()  [unwired: 2 in, 3 out]
          }
          event "eyeFromPx?": Value Change {
            n66 = event-data() -> ()  [unwired: 1 in, 6 out]
            n67 = Enqueue Element(queue=w98, element="eyeFromPx? Changed") -> ()  [unwired: 2 in, 3 out]
          }
          event "alignPR?": Value Change {
            n68 = event-data() -> ()  [unwired: 1 in, 6 out]
            n69 = Enqueue Element(queue=w103, element="alignPR? Changed") -> (queue out=w101:refnum<queue>)  [unwired: 2 in, 2 out]
            n70 = Enqueue Element(queue=w101, element="Set Plot Channels") -> ()  [unwired: 2 in, 3 out]
          }
          event "manualGOff?": Value Change {
            n71 = event-data() -> ()  [unwired: 1 in, 6 out]
            n72 = Enqueue Element(queue=w105, element="ManualGOff? Changed") -> ()  [unwired: 2 in, 3 out]
          }
        }
      }
      frame "DO Process" {
        # "Clear Processing Errors"
        n73 = for {
          tunnel: w108 -> [w111]
          tunnel: string[] ["Check Files", "Load Data", "Get File Info", "Report Errors"] -> [w110] mode=indexing
          n74 = Enqueue Element(queue=w111, element=w110) -> ()  [unwired: 2 in, 3 out]
        }
        n75 = local write "Process Error"(errorcluster {"status"=FALSE, "code"=0, "source"=""} ("Process Error")) -> ()
      }
      frame "Check Files" {
        n76 = local read "Process Error"() -> (w112:errorcluster)
        n77 = case shown="No Error" w112 {
          frame No Error {
            # "Only require head calibration  file when head calibration is selected"
            # "Only require eye calibration file when eye calibration is selected"
            # "Always require data file"
            n78 = local read "Head Calibration File"() -> (w123:path)
            n79 = local read "Eye Calibration File"() -> (w124:path)
            n80 = local read "Data File"() -> (w125:path)
            n81 = local read "eyeFromPx?"() -> (w122:bool)
            n82 = local read "alignPR?"() -> (w120:bool)
            n83 = call <vilib>:"Is Path and Not Empty.vi"("path"=w125) -> ("Is Path and Not Empty?"=w118:bool)  [unwired: 4 in]
            n84 = call <vilib>:"Is Path and Not Empty.vi"("path"=w123) -> ("Is Path and Not Empty?"=w119:bool)  [unwired: 4 in]
            n85 = call <vilib>:"Is Path and Not Empty.vi"("path"=w124) -> ("Is Path and Not Empty?"=w121:bool)  [unwired: 4 in]
            n86 = Compound Arithmetic op=OR(invert w120, w119) -> (w116:bool)
            n87 = Compound Arithmetic op=OR(invert w122, w121) -> (w117:bool)
            n88 = Compound Arithmetic op=AND(w118, w117, w116) -> (w115:bool)
            n89 = case shown="False" w115 {
              tunnel: [errorcluster {"status"=TRUE, "code"=0, "source"="Files must be specified for each selected file field."} ("error constant") _] -> w114
              frame False {
                # "File requirements not met. Error."
              }
              frame True {
                # "All file requirments met."
              }
            }
            n90 = local write "Process Error"(w114) -> ()
          }
          frame Error {
          }
        }
      }
      frame "Load Data" {
        n91 = local read "Head Calibration File"() -> (w149:path)
        n92 = local read "Eye Calibration File"() -> (w150:path)
        n93 = local read "Pitch"() -> (w146:dbl)
        n94 = local read "Yaw"() -> (w145:dbl)
        n95 = local read "Roll"() -> (w147:dbl)
        n96 = local read "manualGOff?"() -> (w148:bool)
        n97 = local read "Process Error"() -> (w138:errorcluster)
        n98 = local read "eyeFromPx?"() -> (w127:bool)
        n99 = local read "Data File"() -> (w151:path)
        n100 = local read "alignPR?"() -> (w129:bool)
        n101 = Build Array(w147, w146, w145) -> (w144:dbl[])
        n102 = Path To String(path=w151) -> (string=w143:string)
        n103 = Path To String(path=w150) -> (string=w142:string)
        n104 = Path To String(path=w149) -> (string=w140:string)
        n105 = Boolean To (0,1)(Boolean=w127) -> (0, 1=w128:i16)
        n106 = Boolean To (0,1)(Boolean=w129) -> (0, 1=w130:i16)
        n107 = Boolean To (0,1)(Boolean=w148) -> (0, 1=w139:i16)
        n108 = script code="%%%%%%%%%%%%%%%%%%%%%%%%%%%%%%%%%%%%%%%%%%%%%%%%%%%%%%\n% EMA SCRIPT\n%%%%%%%%%%%%%%%%%%%%%%%%%%%%%%%%%%%%%%%%%%%%%%%%%%%%%%\n\n%------------------ CALCULATE EYE PX -> DEG TRANSFORM----------------------\nif doEyeFromPxCalc\n    load(eyeCalibPath);\n\n    %---- CALCULATE TRANSFORM PX -> DEG ----\n    % Set eye reference position to centre calibration dot position\n    EPos_Ref = C_left(1,:);\n\n    % Zero calibration points  \n    C_left_zeroed = bsxfun(@minus, C_left, EPos_Ref);\n\n    % Solve for transform T\n    % Note Linear Transform Assumption: Pos_deg = Pos_px * T\n    Te = pinv(C_left_zeroed)*[0 0; 0 -8.5; 0 8.5; -8.5 0; 8.5 0];\nend\n\n%-------------------------- GET GYRO OFFSET -------------------------------\nif useManualGyroOffset\n    HVel_Ref = manualGyroOffset;\nelse\n    % Older eye cal files do not have sensor_velo_median\n    try\n        HVel_Ref = sensor_velo_median;\n    catch\n        HVel_Ref = [0 0 0];\n    end\nend\n\n%--------------- CALCULATE HEAD PITCH/ROLL AXIS ALIGNMENT -----------------\nif doHeadCal\n    % Get head pitch velocities from head calibration recording\n    load(headCalibPath);\n    HVelc = Data(:, strmatch('HeadInertialVel', DataNames));\n\n    % Zero gyro\n    HVelc = bsxfun(@minus, HVelc, HVel_Ref);\n\n    % Only use Roll and Pitch Data for calibration. Yaw Axis is correct.\n    HVelRP = HVelc(:,1:2);\n    \n    %Use only the fastest 75% to ensure actual pitching data is being used\n    HvSum = sum(abs(HVelRP), 2);\n    headVelThresh = prctile(HvSum, 75); \n\n    % Calculate instantaneous angle between Expected Direction and File Pitching\n    a = nan(1, length(HVelRP));\n    for i = 1:length(HVelRP)\n        % Do not do calculations for low velocity or NaN data\n        if isnan(HvSum)\n            continue\n        elseif HvSum(i) <= headVelThresh\n            continue\n        end\n        \n        % Determine angle based on atan2 method:\n        % a = atan2d(x1*y2-y1*x2,x1*x2+y1*y2); V1 = Pitch = [0, 1], V2 = HVelRP(i)\n        a(i) = atan2d(-HVelRP(i,1), HVelRP(i,2));\n\n        % Make sure the transform gives pitch +ve downwards\n        if a(i) > 0 \n            a(i) = a(i) - 180;\n        end\n    end\n\n    % Calculate general angle between Expected Pitch Direction and File Pitching\n    A = nanmedian(a);\n   \n    % Calculate Head calibration transform\n    A = -A; % We want to undo the rotation so negate the angle.\n    Th = [cosd(A), -sind(A), 0; sind(A), cosd(A), 0; 0, 0, 1];\n    \nelse\n    % Identity matrix to specify no transform.\n    Th = eye(3);\nend\n\n%------------------------ CALCULATE REC FILE DATA -------------------------\nload(dataPath);\n\n%---- HEAD DATA ----\n%Load from file\nHVel = Data(:, strmatch('HeadInertialVel', DataNames));\n\n%Apply calibration\nHVel = bsxfun(@minus, HVel, HVel_Ref);  % Zero                                           \nHVel = (Th * HVel')';                   % Rotate pitch/roll axes\n\n%Calculate LARP/RALP\nHVelLR = HVel * [cosd(-45), -sind(-45), 0; sind(-45), cosd(-45), 0; 0, 0, 1];\nHVelLR = HVelLR(:, 1:2);\n\n%---- EYE DATA ----\nif doEyeFromPxCalc\n    %Load from file\n    EPosPx = Data(:, [strmatch('LeftPupilCol', DataNames),...\n        strmatch('LeftPupilRow', DataNames)]);\n    \n    %Calculate eye position from pupil pixel centoroid\n    EPosPx_zeroed = bsxfun(@minus, EPosPx, EPos_Ref);   % Zero\n    EPos = EPosPx_zeroed*Te;                            % Px -> Deg\n    EPos(:, 1) = EPos(:, 1) ./ cosd(EPos(:, 2));        % Correct yaw to match Fick System (ADDED: 17/01/2017)\n    EPos = [EPos(:, 2), EPos(:, 1)];                    % Swap to Pitch-Yaw convention\n    \n    % Calculate Eye Velocity...\n    % 1D differentiation used to calculate velocity due to the lack of torsion\n    % information. Gradient function used for central differentiation routine.\n    EVel_pitch = gradient(EPos(:,1), 1/SamplingRate);\n    EVel_yaw = gradient(EPos(:,2), 1/SamplingRate);\n    EVel = [EVel_pitch, EVel_yaw];\nelse\n    %Load from file\n    EPos = Data(:, [strmatch('LeftEyeVer', DataNames),...\n        strmatch('LeftEyeHor', DataNames)]);\n    EVel = Data(:, [strmatch('LeftEyeVelY', DataNames),...\n        strmatch('LeftEyeVelZ', DataNames)]);\nend\n\n%-------------------------- OUTPUT TO LABVIEW -----------------------------\nDataLength = length(HVel);\nDataOut = nan(24,DataLength);\nDataOut(2, :) = HVel(:, 3)';         % Head Velocity Yaw\nDataOut(4, :) = HVel(:, 2)';         % Head Velocity Pitch\nDataOut(6, :) = HVel(:, 1)';         % Head Velocity Roll\nDataOut(7:8, :) = HVelLR';          % Head Velocity (LARP-RALP)\nDataOut(10:11, :) = EPos';          % Eye Position (Pitch-Yaw)\nDataOut(13:14, :) = EVel';           % Eye Velocity (Pitch-Yaw)\n\n%---- OTHER LABVIEW PARAMETERS ----\nStimulus = strcat('HIT-', Condition);\n\n%%%%%%%%%%%%%%%%%%%%%%%%%%%%%%%%%%%%%%%%%%%%%%%%%%%%%%\n%END\n%%%%%%%%%%%%%%%%%%%%%%%%%%%%%%%%%%%%%%%%%%%%%%%%%%%%%%" ("Load patient name and data")("??"=w138, "dataPath"=w143, "doEyeFromPxCalc"=w128, "eyeCalibPath"=w142, "headCalibPath"=w140, "doHeadCal"=w130, "manualGyroOffset"=w144, "useManualGyroOffset"=w139) -> ("??"=w141:errorcluster, "Subject"=w135:string, "Examinator"=w134:string, "DataOut"=w133:dbl[][], "SamplingRate"=w132:dbl, "Stimulus"=w131:string)
        n109 = case shown="No Error" w141 {
          selector: w141 -> [_ w162]
          tunnel: w137 -> [w158 w159]
          tunnel: [w157 w159] -> w136
          tunnel: w135 -> [w156 _]
          tunnel: w134 -> [w155 _]
          tunnel: w133 -> [w154 _]
          tunnel: w132 -> [w153 _]
          tunnel: w131 -> [w152 _]
          frame No Error {
            n110 = Bundle By Name(cluster=w158, "Experiment Parameters 2.Subject"=w156, "Experiment Parameters 2.Experimenter"=w155, "Data File.Data Channels"=w154, "Data File.Sample Rate"=w153, "Experiment Parameters.Stimulus"=w152) -> (w157:T3)
          }
          frame Error {
            n111 = Merge Errors(errorcluster {"status"=TRUE, "code"=0, "source"="Unable to parse the selected files. Check that the selected files are correct and that MATLAB is installed and licensed on this computer."} ("error in"), w162) -> (w161:errorcluster)
            n112 = local write "Process Error"(w161) -> ()
          }
        }
      }
      frame "Get File Info" {
        n113 = local read "Process Error"() -> (w165:errorcluster)
        n114 = case shown="No Error" w165 {
          tunnel: w164 -> [w168 w173]
          tunnel: [w169 w173] -> w163
          frame No Error {
            # "Valid Files"
            n115 = local read "Eye Calibration File"() -> (w166:path)
            n116 = local read "Data File"() -> (w167:path)
            n117 = Strip Path(path=w167) -> (stripped path=w172:path, name=w171:string)
            n118 = Strip Path(path=w166) -> (name=w170:string)  [unwired: 1 out]
            n119 = Bundle By Name(cluster=w168, "Experiment data path"=w172, "filename"=w171, "calibration name"=w170) -> (w169:T3)
          }
          frame Error {
          }
        }
      }
      frame "Report Errors" {
        n120 = local read "Process Error"() -> (w175:errorcluster)
        n121 = call <vilib>:"Simple Error Handler.vi"("error in (no error)"=w175) -> ("error out"=w177:errorcluster)  [unwired: 4 in, 4 out]
        n122 = case shown="No Error" w175 {
          tunnel: w174 -> [w180 _]
          frame No Error {
            # "Processing was a success. We can save the results and close this dialog."
            n123 = Enqueue Element(queue=w180, element="Exit") -> ()  [unwired: 2 in, 3 out]
          }
          frame Error {
            # "Processing was not a success. Do nothing to return to the Idle state."
          }
        }
        n124 = call <vilib>:"Clear Errors.vi"("error in (no error)"=w177) -> ("error out"=w176:errorcluster)  [unwired: 5 in, 1 out]
        n125 = local write "Process Error"(w176) -> ()
      }
      frame "Find Calibration" {
        # "No longer used. It was causing trouble selecting the wrong calibration file and didn't work frequently enough to not be confusing."
        n126 = disable-structure shown="Disabled" {
          frame Disabled {
            n127 = local read "Eye Calibration File"() -> (w184:path)
            n128 = call <vilib>:"Is Path and Not Empty.vi"("path"=w184) -> ("Is Path and Not Empty?"=w183:bool)  [unwired: 4 in]
            n129 = case shown="False" w183 {
              tunnel: [w186 w196] -> w182
              tunnel: w184 -> [_ w196]
              frame False {
                # "Search file directory for calibration files."
                # "Valid calibration not specified. Find one."
                n130 = local read "Data File"() -> (w185:path)
                n131 = Strip Path(path=w185) -> (stripped path=w191:path)  [unwired: 1 out]
                n132 = List Folder(path=w191, pattern="p?????s???_calib.mat") -> (path out=w187:path, filenames=w188:string[])  [unwired: 2 in, 2 out]
                n133 = Empty Array?(array=w188) -> (empty?=w189:bool)
                n134 = case shown="False" w189 {
                  tunnel: w188 -> [w195 _]
                  tunnel: w187 -> [w194 _]
                  tunnel: [w192 _] -> w186
                  frame False {
                    # "The array is already sorted alphabetically."
                    # "Found calibration files. Get latest one."
                    n135 = Delete From Array(array=w195) -> (deleted portion=w193:string)  [unwired: 2 in, 1 out]
                    n136 = Build Path(base path=w194, name or relative path=w193) -> (appended path=w192:path)
                  }
                  frame True {
                    # "Did not find calibration files. Do nothing."
                  }
                }
              }
              frame True {
                # "Calibration already specified manually."
              }
            }
            n137 = local write "Eye Calibration File"(w182) -> ()
          }
          frame Enabled {
          }
        }
      }
      frame "Exit" {
        n138 = local write "Cancelled"(FALSE ("Cancelled")) -> ()
      }
      frame "Exit without Save" {
        n139 = local write "Cancelled"(TRUE) -> ()
      }
    }
  }
  "Data OUT" <- w2
  n140 = disable-structure shown="Disabled" {
    frame Disabled {
      # "LEGACY CODE"
      n141 = stacked-sequence {
        frame #0 {
          # "Original Load Script -> Loads Data Straight From File -> Used with pototype EyeSeeCam"
          n142 = script code="%Load file\nload(filePath);\n\n%Generate stimulus name\nStimulus = strcat('HIT-', Condition);\n\n%Create DataOut matrix\n[dataLength, ~] = size(Data);\nDataOut = zeros(24, dataLength);\n\n%Load velocity data and check for data which has not been captured\nPositions = [2, 4, 6, 12, 13, 14, 20, 21, 22];\nNames = {'HeadInertialVelZ', 'HeadInertialVelY', 'HeadInertialVelX', ...\n    'LeftEyeVelX', 'LeftEyeVelY', 'LeftEyeVelZ', ...\n    'RightEyeVelX', 'RightEyeVelY', 'RightEyeVelZ'};\nfor i = 1:length(Positions)\n    d = Data(:, strmatch(Names{i}, DataNames))';\n    if ~isempty(d)\n        DataOut(Positions(i), :) = d;\n    end\nend\n\n%Calculate  RALP and LARP for Head\nR = rotz(-45);\nHeadRot = R*[DataOut(6,:); DataOut(4,:); DataOut(2,:)];\nDataOut(7, :) = HeadRot(2,:);   %Hl\nDataOut(8, :) = HeadRot(1,:);   %Hr\n\n%If HIT was 3D calculate eye RALP and LARP in the same way\n%If HIT was 2D both RALP and LARP = Pitch\nif HITdim == 1\n     %3D Head Impulse\n     LEyeRot = R*[DataOut(12,:); DataOut(13,:); DataOut(14,:)];\n     REyeRot = R*[DataOut(20,:); DataOut(21,:); DataOut(22,:)];\n     DataOut(15, :) = LEyeRot(2,:);    %Ll\n     DataOut(16, :) = LEyeRot(1,:);    %Lr\n     DataOut(23, :) = REyeRot(2,:);    %Rl\n     DataOut(24, :) = REyeRot(1,:);    %Rr\nelse\n     %2D Head Impulse\n     DataOut(15,:) = DataOut(13,:);   %Ll = Ly\n     DataOut(16,:) = DataOut(13,:);   %Lr = Ly\n     DataOut(23,:) = DataOut(21,:);   %Rl = Ry\n     DataOut(24,:) = DataOut(21,:);   %Rr = Ry\nend" ("Load patient name and data")() -> ()  [unwired: 3 in, 6 out]
        }
        frame #1 {
          # "Second Load Script -> Calculates Eye Velocity from pixel position -> Used with Interacoustics commercial EyeSeeCam"
          n143 = script code="%---- LOAD DATA ----\nload(calibPath);\nload(dataPath);\n\n%---- CALCULATE TRANSFORM PX -> DEG ----\n% Note: Pos_deg = Pos_px * T\nLeftPupilPx_zeroed = bsxfun(@minus,LeftPupilPx,C_left(1,:));\nC_left_zeroed = bsxfun(@minus,C_left,C_left(1,:));\nT = pinv(C_left_zeroed)*[0 0; 0 -8.5; 0 8.5; -8.5 0; 8.5 0];\n\n%---- GET DATA FROM RECORDING FILE USING NAMES ----\nHVel = Data(:, strmatch('HeadInertialVel', DataNames));\nEPosPx = Data(:, [strmatch('LeftPupilCol', DataNames), strmatch('LeftPupilRow', DataNames)]);\n\n%---- CALCULATE RALP AND LARP HEAD VELOCITY ----\nHVelRL = HVel*rotz(-45);\nHVelRL = HVelRL(:, 1:2);\n\n%---- CALCULATE EYE POSITION (DEG) FROM CoM PIXEL POSITION ----\nPos_deg = EPosPx*T;\nPos_deg = [zeros(length(Pos_deg), 1), Pos_deg(:, 2), Pos_deg(:, 1)];\n\n%---- CALCULATE EYE VELOCITY (DEG/S) ----\n%Calculate fick angle time differential\ndAdt = diff(Pos_deg, 1, 1) * SamplingRate;\n\n%Shorten fick angle vector to match differential length\nPos_deg = Pos_deg(1:end-1, :);\n\n%Calculate angular velocity according to Goldstein, 1980 method\nVel_deg = [...\n    dAdt(:, 1).*cosd(Pos_deg(:, 3)).*cosd(Pos_deg(:, 2)) - dAdt(:, 2).*sind(Pos_deg(:, 3)),...\n    dAdt(:, 1).*sind(Pos_deg(:, 3)).*cosd(Pos_deg(:, 2)) + dAdt(:, 2).*cosd(Pos_deg(:, 3)),...\n    dAdt(:, 3) - dAdt(:, 1).*sind(Pos_deg(:, 2))...\n    ];\n\n%---- CALCULATE RALP AND LARP EYE VELOCITY (DEG/S) ----\nif HITtype == 0\n    % 2D Type\n    EVelRL = [Vel_deg(:, 2), Vel_deg(:, 2)];\nelse \n    %3D Type\n     EVelRL = Vel_deg*rotz(-45);\n     EVelRL = EVelRL(:, 1:2);\nend\n\n%---- OUTPUT LABVIEW DATA ----\nDataLength = length(Pos_deg);\nDataOut = nan(24,DataLength);\nDataOut(2, :) = HVel(1:DataLength, 3)';\nDataOut(4, :) = HVel(1:DataLength, 2)';\nDataOut(6, :) = HVel(1:DataLength, 1)';\nDataOut(7, :) = HVelRL(1:DataLength, 2)';\nDataOut(8, :) = HVelRL(1:DataLength, 1)';\nDataOut(9:11, :) = Pos_deg(1:DataLength, :)';\nDataOut(12:14, :) = Vel_deg(1:DataLength, :)';\nDataOut(15, :) = EVelRL(1:DataLength, 2)';\nDataOut(16, :) = EVelRL(1:DataLength, 1)';\n\n%---- OUTPUT OTHER LABVIEW PARAMETERS ----\nStimulus = strcat('HIT-', Condition);" ("Load patient name and data")() -> ()  [unwired: 4 in, 6 out]
        }
        frame #2 {
          # "Third Load Script -> Included head pitch/yaw axis alignment"
          n144 = script code="%%%%%%%%%%%%%%%%%%%%%%%%%%%%%%%%%%%%%%%%%%%%%%%%%%%%%%%%%%%%\n% EMA SCRIPT...\n%%%%%%%%%%%%%%%%%%%%%%%%%%%%%%%%%%%%%%%%%%%%%%%%%%%%%%%%%%%%\n\n%------------------------------- EYE CALIBRATION -----------------------------\nload(calibPath);\n\n%---- CALCULATE TRANSFORM PX -> DEG ----\n% Set eye reference position to centre calibration dot position\nEPos_Ref = C_left(1,:);\n\n% Zero calibration points  \nC_left_zeroed = bsxfun(@minus, C_left, EPos_Ref);\n\n% Solve for transform T\n% Note Linear Transform Assumption: Pos_deg = Pos_px * T\nTe = pinv(C_left_zeroed)*[0 0; 0 -8.5; 0 8.5; -8.5 0; 8.5 0];\n\n%--------------------------- HEAD CALIBRATION -----------------------------\n\n% Get gyro offset from _calib file if not provided manually\nif ManualHVel_Ref == 0\n    HVel_Ref = sensor_velo_median;\nend\n\n% Do Pitch / Roll Axis alignment if head movement is expected to be 3D\nif HITtype == 1\n    % Get head pitch velocities from head calibration recording\n    load(headCalibPath);\n    HVelc = Data(:, strmatch('HeadInertialVel', DataNames));\n\n    % Zero gyro\n    HVelc = bsxfun(@minus, HVelc, HVel_Ref);\n\n    % Only use Roll and Pitch Data for calibration. Yaw Axis is correct.\n    HVelRP = HVelc(:,1:2);\n\n    % Calculate instantaneous angle between Expected Direction and File Pitching\n    a = nan(1, length(HVelRP));\n    for i = 1:length(HVelRP)\n        % Do not do calculations for low velocity or NaN data:\n        HvSum = sum(abs(HVelRP(i,1:2)));\n        if HvSum <= headVelThresh || isnan(HvSum)\n            continue\n        end\n\n        % Determine angle based on atan2 method:\n        % a = atan2d(x1*y2-y1*x2,x1*x2+y1*y2); V1 = Pitch = [0, 1], V2 = HVelRP(i)\n        a(i) = atan2d(-HVelRP(i,1), HVelRP(i,2));\n\n        % Make sure the transform gives pitch +ve downwards\n        if a(i) > 0 \n            a(i) = a(i) - 180;\n        end\n    end\n\n    % Calculate general angle between Expected Pitch Direction and File Pitching\n    A = nanmedian(a);\n\n    % Calculate Head calibration transform\n    Th = rotz(-A);\nend\n\n%---------------------------- RECORDING DATA ------------------------------\nload(dataPath);\n\n%---- GET DATA FROM RECORDING FILE USING NAMES ----\nHVel = Data(:, strmatch('HeadInertialVel', DataNames));\nEPosPx = Data(:, [strmatch('LeftPupilCol', DataNames), strmatch('LeftPupilRow', DataNames)]);\n\n%---- APPLY HEAD VELOCITY CALIBRATION ----\nHVel = bsxfun(@minus, HVel, HVel_Ref);  % Zero\nif HITtype == 1                                              \n    HVel = (Th * HVel')';                                  % Rotate using head cal result to align pitch/roll axes      \nend\n\n%---- CALCULATE LARP AND RALP HEAD VELOCITY ----\nHVelLR = HVel*rotz(-45);\nHVelLR = HVelLR(:, 1:2);\n\n%---- CALCULATE EYE POSITION (DEG) FROM PIXEL POSITION ----\nEPosPx_zeroed = bsxfun(@minus, EPosPx, EPos_Ref);   % Zero\nEPos = EPosPx_zeroed*Te;                            % Px -> Deg\nEPos(:, 1) = EPos(:, 1) ./ cosd(EPos(:, 2));     % Correct yaw to match Fick System (ADDED: 17/01/2017)\n\n%Swap from Yaw-Pitch to Pitch-Yaw convention to match the head data\nEPos = [EPos(:, 2), EPos(:, 1)];\n\n%---- CALCULATE EYE VELOCITY (DEG/S) ----\n% 1D differentiation used to calculate velocity due to the lack of torsion\n% information. Gradient function used for central differentiation routine.\nEVel_pitch = gradient(EPos(:,1), 1/SamplingRate);\nEVel_yaw = gradient(EPos(:,2), 1/SamplingRate);\nEVel = [EVel_pitch, EVel_yaw];\n\n%-------------------------- OUTPUT TO LABVIEW -----------------------------\nDataLength = length(HVel);\nDataOut = nan(24,DataLength);\nDataOut(2, :) = HVel(:, 3)';         % Head Velocity Yaw\nDataOut(4, :) = HVel(:, 2)';         % Head Velocity Pitch\nDataOut(6, :) = HVel(:, 1)';         % Head Velocity Roll\nDataOut(7:8, :) = HVelLR';          % Head Velocity (LARP-RALP)\nDataOut(10:11, :) = EPos';          % Eye Position (Pitch-Yaw)\nDataOut(13:14, :) = EVel';           % Eye Velocity (Pitch-Yaw)\n\n%---- OTHER LABVIEW PARAMETERS ----\nStimulus = strcat('HIT-', Condition);" ("Load patient name and data")() -> ()  [unwired: 8 in, 6 out]
        }
      }
    }
    frame Enabled {
    }
  }
